vi "Sensor State Indicators.vi"() -> ()   [LabVIEW 2013]
panel:
  out "Z Position":dbl
  out "Y Position":dbl
  out "X Position":dbl
  out "Signal Deviation From Center":dbl
  out "Signal Strength":dbl
  # "Position"
  # "Z"
  # "Y"
  # "X"
  # "Signal"
  # "Deviation"
  # "Strength"
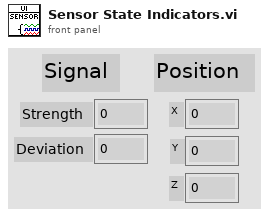
[diagram p1: front panel]
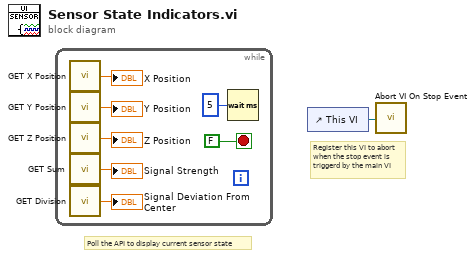
[diagram p0: block diagram]
diagram:
  # "Register this VI to abort\nwhen the stop event is\ntriggerd by the main VI"
  # "Poll the API to display current sensor state"
  n1 = while {
    stop <- FALSE stop-if-true
    n2 = call "GET X Position.vi"() -> ("X Position"=→"X Position":dbl)
    n3 = call "GET Y Position.vi"() -> ("Y Position"=→"Y Position":dbl)
    n4 = call "GET Z Position.vi"() -> ("Z Position"=→"Z Position":dbl)
    n5 = call "GET Sum.vi"() -> ("Sum"=→"Signal Strength":dbl)
    n6 = call "GET Division.vi"() -> ("Division"=→"Signal Deviation From Center":dbl)
    n7 = Wait (ms)(milliseconds to wait=u32 5) -> ()  [unwired: 1 out]
  }
  n8 = control-ref of="This VI"() -> (w1:refnum<vi>)
  n9 = call "Abort VI On Stop Event.vi"("VI Reference"=w1) -> ()
